vi "FormatClass.vi"(5 "type":T1, 6 "name":string, 7 "parameters/ancestors":string[](array[string])=["self"], 9 "body":string[](array[string])) -> (3 "python":string)   [LabVIEW 2014, in "Python Functions.lvlib"]
uses:
  Python Functions.lvlib
  ClassTypeTD.ctl
  ListTypesTD.ctl
  <vilib>/Utility/error.llb/whitespace.ctl
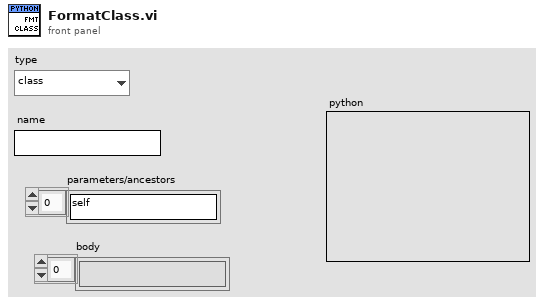
[diagram p1: front panel]
types:
  T1 = typedef "Python Functions.lvlib/ClassTypeTD.ctl" = enum16{"class", "function"}
  T2 = typedef "whitespace.ctl" = u16
  T3 = typedef "Python Functions.lvlib/ListTypesTD.ctl" = enum16{"list", "tuple", "parameter list", "output list"}
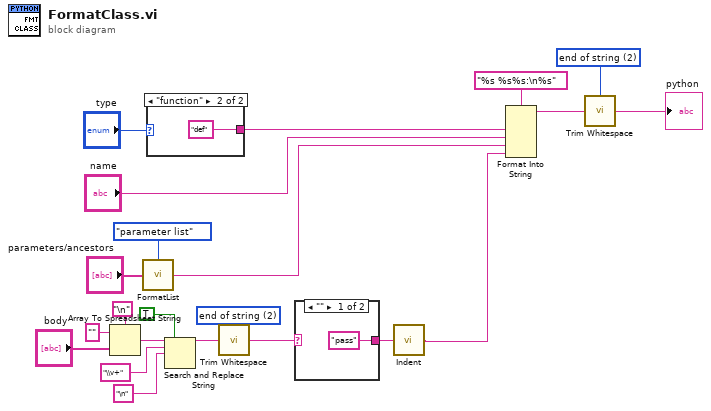
[diagram p0: block diagram]
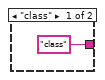
[diagram p3: hidden frame]
diagram:
  w6 = T2 2 items=["both", "start of string", "end of string"] ("location (both)")
  w13 = T2 2 items=["both", "start of string", "end of string"] ("location (both)")
  n1 = Array To Spreadsheet String(delimiter (Tab)="\n", array="body", 3:"" ("format string")) -> (spreadsheet string=w5:string)
  n2 = call "FormatList.vi"("values"="parameters/ancestors", "type"=ListTypesTD."parameter list") -> ("python object"=w17:string)
  n3 = case shown="\"function\"" "type" {
    tunnel: ["class" "def"] -> w21
    frame "class" {
    }
    frame "function" {
    }
  }
  n4 = Search and Replace String(replace all?=TRUE ("replace all? (F)"), input string=w5, search string="\\v+", replace string="\n" ("replace string (\"\")")) -> (result string=w4:string)  [unwired: 4 in, 3 out]
  n5 = call <vilib>:"Trim Whitespace.vi"("string"=w4, "location (both)"=w13) -> ("trimmed string"=w12:string)
  n6 = case shown="\"\"" w12 {
    selector: w12 -> [_ w26]
    tunnel: ["pass" w26] -> w11
    frame "" {
    }
    frame Default {
    }
  }
  n7 = call "Indent.vi"("string in"=w11) -> ("string out"=w8:string)  [unwired: 1 in]
  n8 = Format Into String(format string="%s %s%s:\n%s", w21, "name", w17, w8) -> (resulting string=w9:string)  [unwired: 2 in, 1 out]
  n9 = call <vilib>:"Trim Whitespace.vi"("string"=w9, "location (both)"=w6) -> ("trimmed string"=→"python":string)
